vi "Set_Instruments.vi"(8 "error in (no error)":errorcluster caption="entrée d'erreur (pas d'erreur)", 10 "Instruments":T1(array[cluster]), 11 "Popup Autotest (Default) en entrée":refnum<class "Popup Autotest (Default).lvclass">) -> (0 "error out":errorcluster caption="sortie d'erreur", 3 "Popup Autotest (Default) en sortie":refnum<class "Popup Autotest (Default).lvclass">)   [LabVIEW 2020, in "Library Instrument & Equipement.lvlib" / "Library Popup.lvlib" / "Popup Autotest (Default).lvclass"]
uses:
  Popup Autotest (Default).lvclass
  Instrument/Instrument (Default)/Class Instrument (Default).lvclass
  Popup Autotest (Default).lvclass/Popup Autotest (Default).ctl
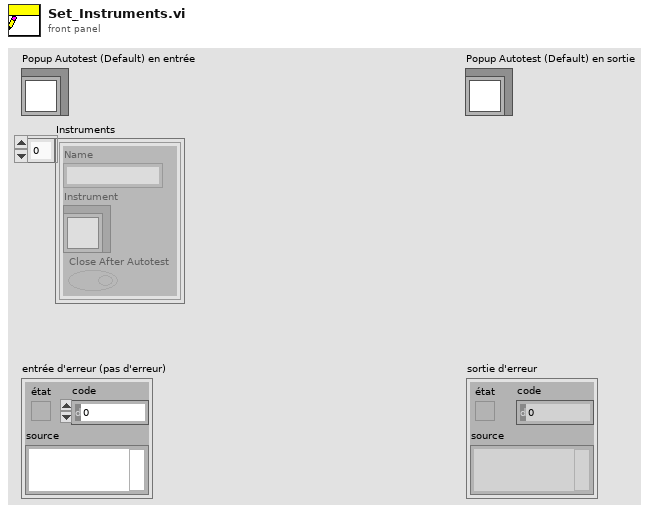
[diagram p1: front panel]
types:
  T1 = cluster{"Name":string, "Instrument":refnum<class "Class Instrument (Default).lvclass">, "Close After Autotest":bool}[]
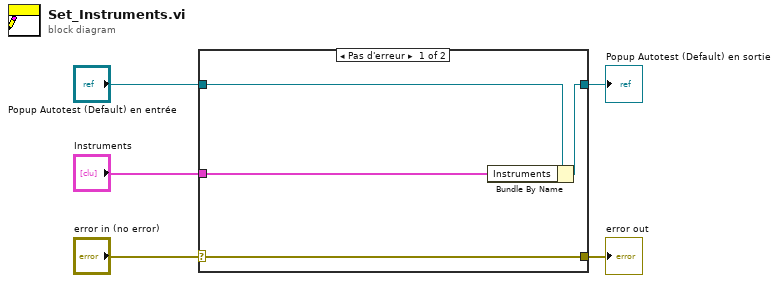
[diagram p0: block diagram]
diagram:
  n1 = case shown="Pas d'erreur" "error in (no error)" {
    selector: "error in (no error)" -> [w9 w10]
    tunnel: [w9 w10] -> w4
    tunnel: [w7 w11] -> w2
    tunnel: "Popup Autotest (Default) en entrée" -> [w8 w11]
    tunnel: "Instruments" -> [w6 _]
    frame No Error {
      n2 = Bundle By Name(cluster=w8, "Instruments"=w6) -> (w7:refnum<class "Popup Autotest (Default).lvclass">)
    }
    frame Error {
    }
  }
  "error out" <- w4
  "Popup Autotest (Default) en sortie" <- w2
